vi "TSM SSC Digital Select Function.vi"(0 "Digital TSM In":T2, 5 "Function":T1=1100 items=["Digital"=1100, "PPMU"=1101, "Off"=1102, "Disconnect"=1103], 11 "error in":errorcluster) -> (4 "Digital TSM Out":T2, 15 "error out":errorcluster)   [LabVIEW 2019]
doc: "Specifies whether digital pattern instruments connected to the specified pin(s) and pin group(s) are controlled by the PPMU, Digital, disconnected, or off. Changes take effect immediately."
uses:
  TSM/TSM SSC Digital.ctl
  <vilib>/NI_TestStand_SemiconductorModule/NI_TestStand_Semiconductor_Module.lvlibp/PinMap/Digital Pattern/PinQueryContext/DigitalPatternPinQueryContext.lvclass
  SSC Digital/SSC Digital.ctl
  <instrlib>/niDigital/niDigital.llb/niDigital Selected Function.ctl
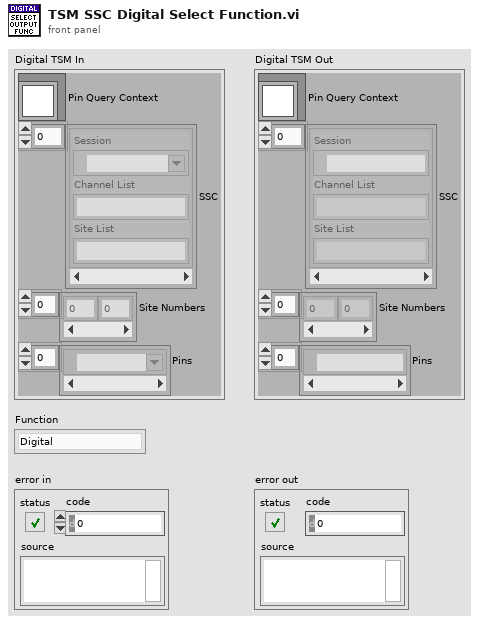
[diagram p1: front panel]
types:
  T1 = typedef "niDigital Selected Function.ctl" = i32
  T2 = typedef "TSM SSC Digital.ctl" = cluster{"Pin Query Context":refnum<class "DigitalPatternPinQueryContext.lvclass">, "SSC":T3[], "Site Numbers":i32[], "Pins":tag[]}
  T3 = typedef "SSC Digital.ctl" = cluster{"Session":refnum<k15>, "Channel List":string, "Site List":string}
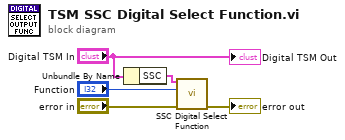
[diagram p0: block diagram]
diagram:
  n1 = Unbundle By Name("Digital TSM In") -> ("SSC"=w4:T3[])
  n2 = call "SSC Digital Select Function.vi"("Digital SSC in"=w4, "Function"="Function", "error in"="error in") -> ("error out"=→"error out":errorcluster)  [unwired: 11 in, 1 out]
  "Digital TSM Out" <- "Digital TSM In"
